vi "Unescape Percent.vi"(8 "error in (no error)":errorcluster, 11 "new error in":T1) -> (0 "error out":errorcluster, 3 "new error out":T1)   [LabVIEW 2016]
uses:
  Error File Management/Controls/NI Error.ctl
  Error File Management/Error File Management.lvlib
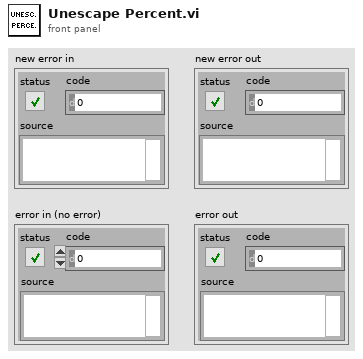
[diagram p1: front panel]
types:
  T1 = typedef "Error File Management.lvlib/NI Error.ctl" = errorcluster
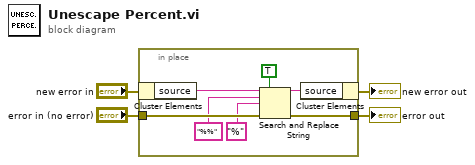
[diagram p0: block diagram]
diagram:
  n1 = in-place {
    in-place-border: "error in (no error)" -> [w8]
    in-place-border: [w7] -> w2
    n2 = in-place-cluster #1("new error in") -> ("source"=w11:string)
    n3 = Search and Replace String(replace all?=TRUE ("replace all? (F)"), input string=w11, search string="%%", replace string="%" ("replace string (\"\")"), error in=w8) -> (result string=w10:string, error out=w7:errorcluster)  [unwired: 3 in, 2 out]
    n4 = in-place-cluster #1("source"=w10) -> (→"new error out":T1)
  }
  "error out" <- w2
